vi "Add element to list (SubVI).vi"(6 "Boolean":bool, 7 "String":refnum<vi>, 9 "Add string":string, 11 "ListBox in":refnum<vi>) -> ()   [LabVIEW 2014]
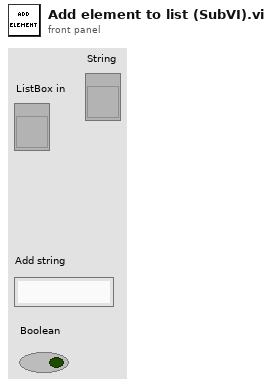
[diagram p1: front panel]
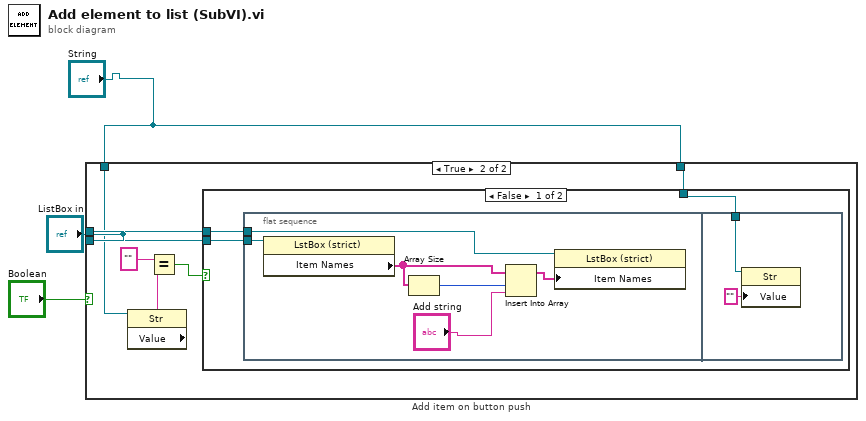
[diagram p0: block diagram]
diagram:
  n1 = case "Add item on button push" shown="True" "Boolean" {
    tunnel: "ListBox in" -> [_ w10]
    tunnel: "ListBox in" -> [_ w9]
    tunnel: "String" -> [_ w8]
    tunnel: "String" -> [_ w4]
    frame False {
    }
    frame True {
      n2 = property on="Property Node" class="Str"(reference=w4) -> ("Value"=w7:string)  [unwired: 1 in, 2 out]
      n3 = Equal?(x="", y=w7) -> (x = y?=w5:bool)
      n4 = case shown="False" w5 {
        tunnel: w10 -> [w13 _]
        tunnel: w9 -> [w12 _]
        tunnel: w8 -> [w11 _]
        frame False {
          n5 = flat-sequence {
            tunnel: w13 -> [w15]
            tunnel: w12 -> [w14]
            tunnel: w11 -> [w20]
            frame #0 {
              n6 = property on="Property Node" class="LstBox (strict)"(reference=w15) -> ("Item Names"=w19:string[])  [unwired: 1 in, 2 out]
              n7 = Array Size(array=w19) -> (size(s)=w16:i32)
              n8 = Insert Into Array(array=w19, index=w16, new element="Add string") -> (w17:string[])
              n9 = property on="Property Node" class="LstBox (strict)"(reference=w14, "Item Names"=w17) -> ()  [unwired: 1 in, 2 out]
            }
            frame #1 {
              n10 = property on="Property Node" class="Str"(reference=w20, "Value"="" ("String")) -> ()  [unwired: 1 in, 2 out]
            }
          }
        }
        frame True {
        }
      }
    }
  }
